vi "Bind to Name - Error Input - Returns Empty String.vi"() -> ()   [LabVIEW 2017, in "JSON Serializable Binder Tests.lvlib"]
uses:
  JSON Serializable Binder Tests.lvlib
  JSON Serializable Binder/JSON Serializable Binder.lvclass
  Fake JSON Serializable/Fake JSON Serializable.lvclass
  <vilib>/Utility/error.llb/Error Cluster From Error Code.vi
  <vilib>/addons/_JKI Toolkits/Caraya/classes/Assert/Assert Equal Value_Variant.vi
  <vilib>/ErrorRing/Error Ring.xnode
  <vilib>/addons/_JKI Toolkits/Caraya/classes/Test/Test.lvclass
  <vilib>/addons/_JKI Toolkits/Caraya/classes/Assert/Assert.lvclass
panel:
  out "error out":errorcluster
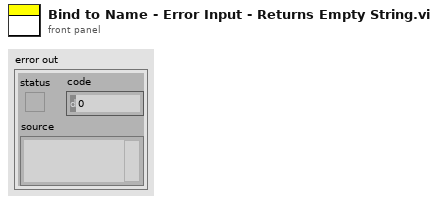
[diagram p1: front panel]
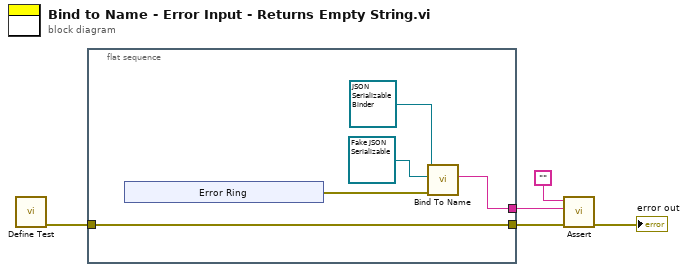
[diagram p0: block diagram]
diagram:
  n1 = call <vilib>:"Define Test.vi"() -> ("error out"=w4:errorcluster)  [unwired: 11 in]
  n2 = flat-sequence {
    tunnel: [w9] -> w5
    tunnel: w4 -> [w9]
    tunnel: [w6] -> w2
    frame #0 {
      n3 = xnode "Error Ring"() -> ("error out"=w10:errorcluster)
      n4 = call-dynamic "Bind To Name.vi"("error in (no error)"=w10, "Type"=refnum<class "Fake JSON Serializable.lvclass"> refnum, "JSON Serializable Binder in"=refnum<class "JSON Serializable Binder.lvclass"> refnum ("JSON Serializable Binder.lvclass")) -> ("Type Name"=w6:string)  [unwired: 6 in, 2 out]
    }
  }
  n5 = call-poly <vilib>:"Assert.vi"("error in (no error)"=w5, "Y"=w2, "X"="") -> ("error out"=→"error out":errorcluster)  [unwired: 8 in]
